vi "Initialize and Configure SLSC SPI.vi"(8 "error in":errorcluster, 11 "SLSC Chip Select DIO Lines":T3) -> (0 "error out":errorcluster, 1 "CS Bits":T4, 2 "SPI API References":T1, 3 "SPI DIO Lines":T2)   [LabVIEW 2014, in "SLSC FPGA Toolkit.lvlib"]
uses:
  SLSC FPGA Toolkit.lvlib
  CD/Source/Shared/SPI Utility/CS Bits.ctl
  SLSC SPI Digital IO Lines.ctl
  <vilib>/SPI API/SPIAPI/DIO/SPI Digital IO Lines.ctl
  <vilib>/SPI API/SPIAPI/Controls/Internal Data (SPI API).ctl
  CD/Source/Shared/SLSC configuration Shared.lvlib
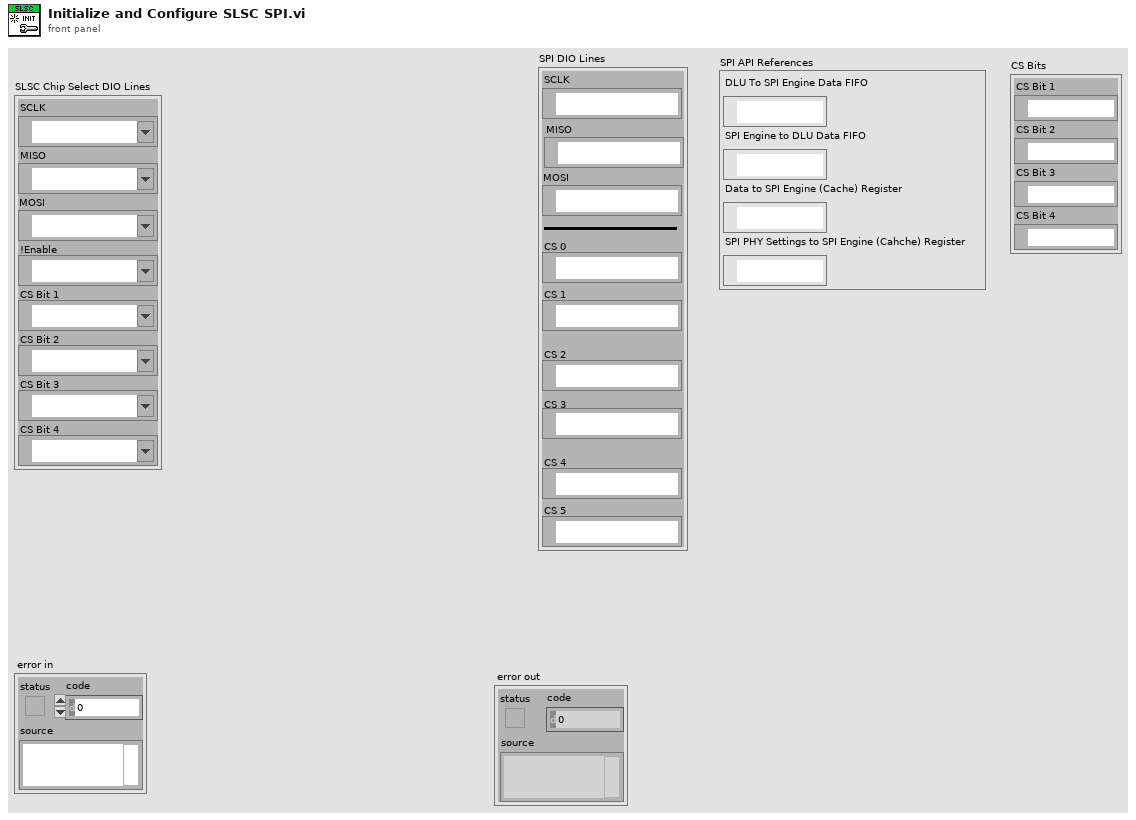
[diagram p1: front panel]
types:
  T1 = typedef "Internal Data (SPI API).ctl" = cluster{"DLU To SPI Engine Data FIFO":refnum<k21>, "SPI Engine to DLU Data FIFO":refnum<k21>, "Data to SPI Engine (Cache) Register":refnum<k21>, "SPI PHY Settings to SPI Engine (Cahche) Register":refnum<k21>}
  T2 = typedef "SPI Digital IO Lines.ctl" = cluster{"SCLK":refnum<k21>, "MISO":refnum<k21>, "MOSI":refnum<k21>, "CS 0":refnum<k21>, "CS 1":refnum<k21>, "CS 2":refnum<k21>, "CS 3":refnum<k21>, "CS 4":refnum<k21>, "CS 5":refnum<k21>}
  T3 = typedef "SLSC FPGA Toolkit.lvlib/SLSC SPI Digital IO Lines.ctl" = cluster{"SCLK":refnum<k21>, "MISO":refnum<k21>, "MOSI":refnum<k21>, "!Enable":refnum<k21>, "CS Bit 1":refnum<k21>, "CS Bit 2":refnum<k21>, "CS Bit 3":refnum<k21>, "CS Bit 4":refnum<k21>}
  T4 = typedef "SLSC configuration Shared.lvlib/CS Bits.ctl" = cluster{"CS Bit 1":refnum<k21>, "CS Bit 2":refnum<k21>, "CS Bit 3":refnum<k21>, "CS Bit 4":refnum<k21>}
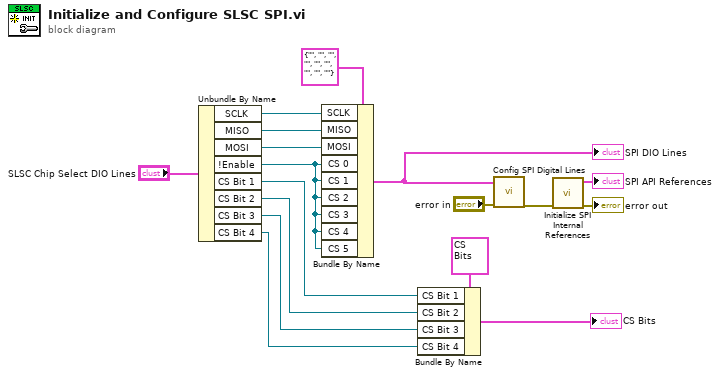
[diagram p0: block diagram]
diagram:
  n1 = Unbundle By Name("SLSC Chip Select DIO Lines") -> ("SCLK"=w14:refnum<k21>, "MISO"=w13:refnum<k21>, "MOSI"=w12:refnum<k21>, "!Enable"=w11:refnum<k21>, "CS Bit 1"=w7:refnum<k21>, "CS Bit 2"=w6:refnum<k21>, "CS Bit 3"=w5:refnum<k21>, "CS Bit 4"=w4:refnum<k21>)
  n2 = Bundle By Name(cluster=T2 {"SCLK"="", "MISO"="", "MOSI"="", "CS 0"="", "CS 1"="", "CS 2"="", "CS 3"="", "CS 4"="", "CS 5"=""} ("Chip Select DIO Lines"), "SCLK"=w14, "MISO"=w13, "MOSI"=w12, "CS 0"=w11, "CS 1"=w11, "CS 2"=w11, "CS 3"=w11, "CS 4"=w11, "CS 5"=w11) -> (w10:T2)
  "SPI DIO Lines" <- w10
  n3 = Bundle By Name(cluster=T4 {"CS Bit 1"="Connector2/DIO3", "CS Bit 2"="Connector2/DIO4", "CS Bit 3"="Connector2/DIO5", "CS Bit 4"="Connector2/DIO6"} ("CS Bits"), "CS Bit 1"=w7, "CS Bit 2"=w6, "CS Bit 3"=w5, "CS Bit 4"=w4) -> (→"CS Bits":T4)
  n4 = call <vilib>:"Config SPI Digital Lines.vi"("error in"="error in", "SPI DIO Lines"=w10) -> ("error out"=w17:errorcluster)  [unwired: 8 in, 1 out]
  n5 = call <vilib>:"Initialize SPI Internal References.vi"("error in"=w17) -> ("error out"=→"error out":errorcluster, "SPI API References"=→"SPI API References":T1)  [unwired: 9 in]
